vi "SLL DE DO Safe Values LV2 Global.vi"(7 "Cases":T2, 8 "error in (no error)":errorcluster, 10 "Value In":bool[](array[boolean]), 11 "Elements In":T1[](array[typedef])) -> (0 "error out":errorcluster, 2 "Value Array Out":bool[](array[boolean]), 3 "Elements Out":T1[](array[typedef]))   [LabVIEW 2013]
uses:
  Controls/SLL DE DO Safe Value Global Options.ctl
  Controls/SLL DE List of Digital Outputs.ctl
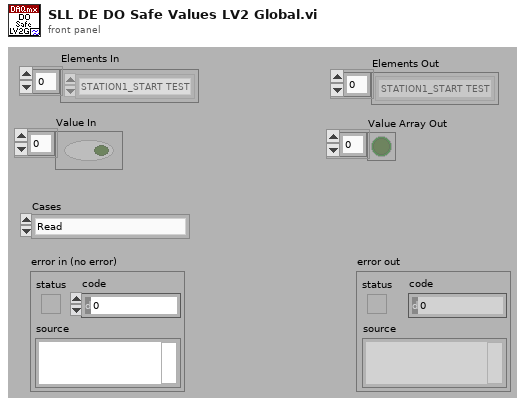
[diagram p1: front panel]
types:
  T1 = typedef "SLL DE List of Digital Outputs.ctl" = enum16{"STATION1_START TEST", "STATION1_STOP TEST", "STATION1_LIGHT1", "STATION1_LIGHT2", "STATION1_LIGHT3", "STATION2_START TEST", "STATION2_STOP TEST", "STATION2_LIGHT1", "STATION2_LIGHT2", "STATION2_LIGHT3", "STATION3_START TEST", "STATION3_STOP TEST", "STATION3_LIGHT1", "STATION3_LIGHT2", "STATION3_LIGHT3", "STATION4_START TEST", "STATION4_STOP TEST", "STATION4_LIGHT1", "STATION4_LIGHT2", "STATION4_LIGHT3"}
  T2 = typedef "SLL DE DO Safe Value Global Options.ctl" = enum16{"Read", "Write"}
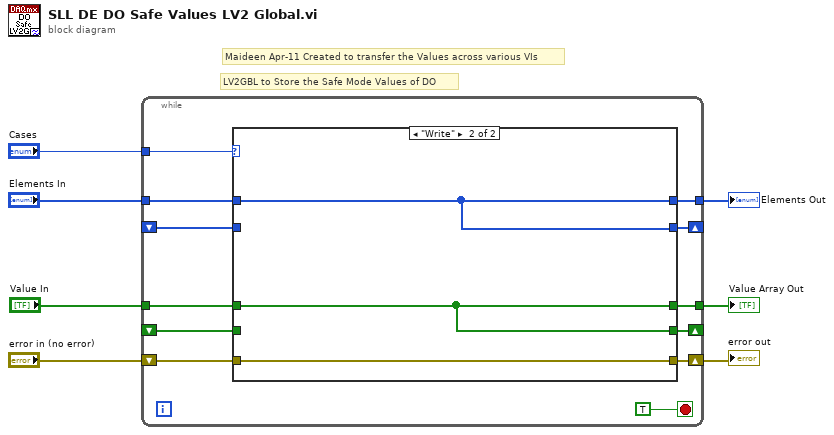
[diagram p0: block diagram]
diagram:
  # "Maideen Apr-11 Created to transfer the Values across various VIs"
  # "LV2GBL to Store the Safe Mode Values of DO"
  n1 = while {
    shift-right: [w18] -> _
    shift-left: _ -> [w17]
    tunnel: "Elements In" -> [w16]
    tunnel: [w15] -> w6
    shift-right: [w13] -> w4
    shift-left: "error in (no error)" -> [w14]
    tunnel: "Value In" -> [w12]
    tunnel: "Cases" -> [w11]
    tunnel: [w10] -> w1
    shift-right: [w9] -> _
    shift-left: _ -> [w8]
    stop <- TRUE stop-if-true
    n2 = case shown="\"Write\"" w11 {
      tunnel: [w21 w25] -> w18
      tunnel: w17 -> [w21 _]
      tunnel: w16 -> [_ w24]
      tunnel: [w21 w25] -> w15
      tunnel: w14 -> [w22 w23]
      tunnel: [w22 w23] -> w13
      tunnel: w12 -> [_ w25]
      tunnel: [w20 w24] -> w10
      tunnel: [w20 w24] -> w9
      tunnel: w8 -> [w20 _]
      frame "Read", Default {
      }
      frame "Write" {
      }
    }
  }
  "error out" <- w4
  "Value Array Out" <- w6
  "Elements Out" <- w1
